vi "Catch.vi"() -> ()   [LabVIEW 2013]
uses:
  CatchEnum.ctl
  DoubleSolenoidAction.ctl
  PnuematicMode.ctl
  Roller States.ctl
panel:
  in  "CatchEnum":T1=enum."Stop"
  out "error out":errorcluster
  in  "error in (no error)":errorcluster
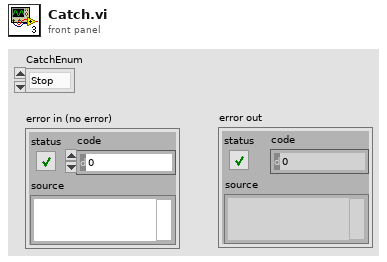
[diagram p1: front panel]
types:
  T1 = typedef "CatchEnum.ctl" = enum16{"Catch", "Stop"}
  T2 = typedef "Roller States.ctl" = enum16{"Off", "Forward", "Reverse"}
  T3 = typedef "PnuematicMode.ctl" = enum16{"Init", "SetState", "Disable"}
  T4 = typedef "DoubleSolenoidAction.ctl" = enum16{"Init", "Middle", "In", "Out"}
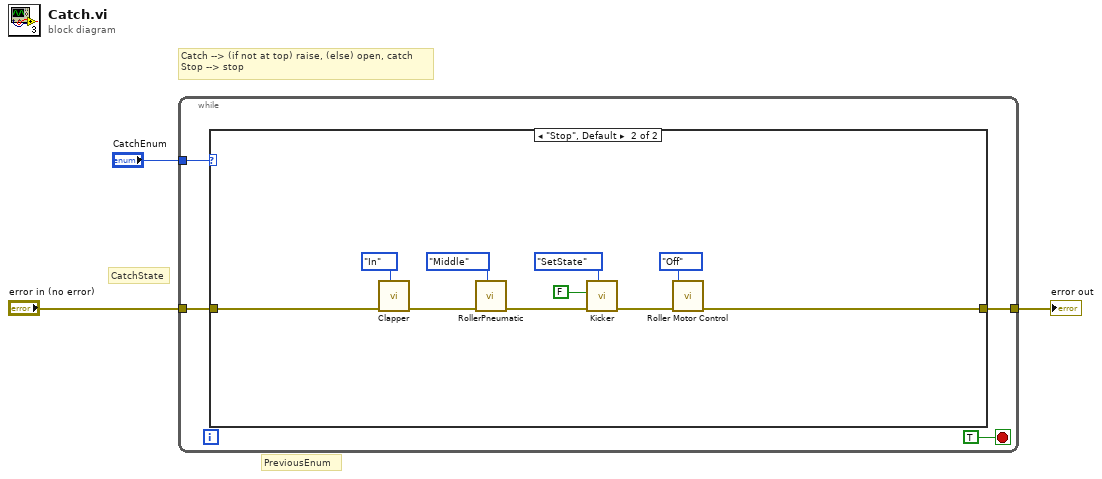
[diagram p0: block diagram]
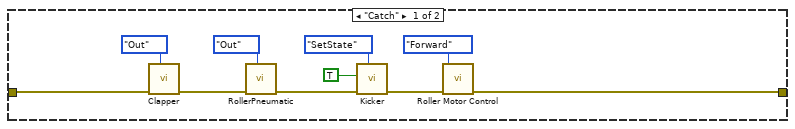
[diagram p2: hidden frame]
diagram:
  # "CatchState"
  # "Catch --> (if not at top) raise, (else) open, catch\nStop --> stop"
  # "PreviousEnum"
  n1 = while {
    tunnel: "error in (no error)" -> [w7]
    tunnel: [w6] -> w2
    tunnel: "CatchEnum" -> [w5]
    stop <- TRUE stop-if-true
    n2 = case shown="\"Stop\", Default" w5 {
      tunnel: w7 -> [w11 w19]
      tunnel: [w8 w18] -> w6
      frame "Catch" {
        n3 = call "Clapper.vi"("State"=DoubleSolenoidAction."Out", "Error in"=w11) -> ("Error out"=w12:errorcluster)  [unwired: 9 in]
        n4 = call "RollerPneumatic.vi"("State"=DoubleSolenoidAction."Out", "Error in"=w12) -> ("Error out"=w13:errorcluster)  [unwired: 9 in]
        n5 = call "Kicker.vi"("Mode"=PnuematicMode."SetState", "error in (no error)"=w13, "State"=TRUE) -> ("error out"=w10:errorcluster)  [unwired: 8 in]
        n6 = call "Roller Motor Control.vi"("Error in"=w10, "RollerState"=Roller_States."Forward") -> ("Error out"=w8:errorcluster)  [unwired: 9 in]
      }
      frame "Stop", Default {
        n7 = call "Clapper.vi"("State"=DoubleSolenoidAction."In", "Error in"=w19) -> ("Error out"=w22:errorcluster)  [unwired: 9 in]
        n8 = call "RollerPneumatic.vi"("State"=DoubleSolenoidAction."Middle", "Error in"=w22) -> ("Error out"=w23:errorcluster)  [unwired: 9 in]
        n9 = call "Kicker.vi"("Mode"=PnuematicMode."SetState", "error in (no error)"=w23, "State"=FALSE) -> ("error out"=w21:errorcluster)  [unwired: 8 in]
        n10 = call "Roller Motor Control.vi"("Error in"=w21, "RollerState"=Roller_States."Off") -> ("Error out"=w18:errorcluster)  [unwired: 9 in]
      }
    }
  }
  "error out" <- w2
